vi "GD_GWID5S_info.vi"(8 "error in (no error)":errorcluster, 10 "glue_id":string, 11 "DBlink":string="Driver={ODBC Driver 17 for SQL Server};Server=localhost\\SQLEXPRESS;Database=ZDX201;UID=labview;PWD=Dsa@54137926") -> (0 "error out":errorcluster)   [LabVIEW 2019]
uses:
  <vilib>/addons/database/Connection.llb/DB Tools Open Connec (String).vi
  <vilib>/addons/database/NI_Database_API.lvlib
panel:
  out "Command 2":string="WHERE [id]=13"
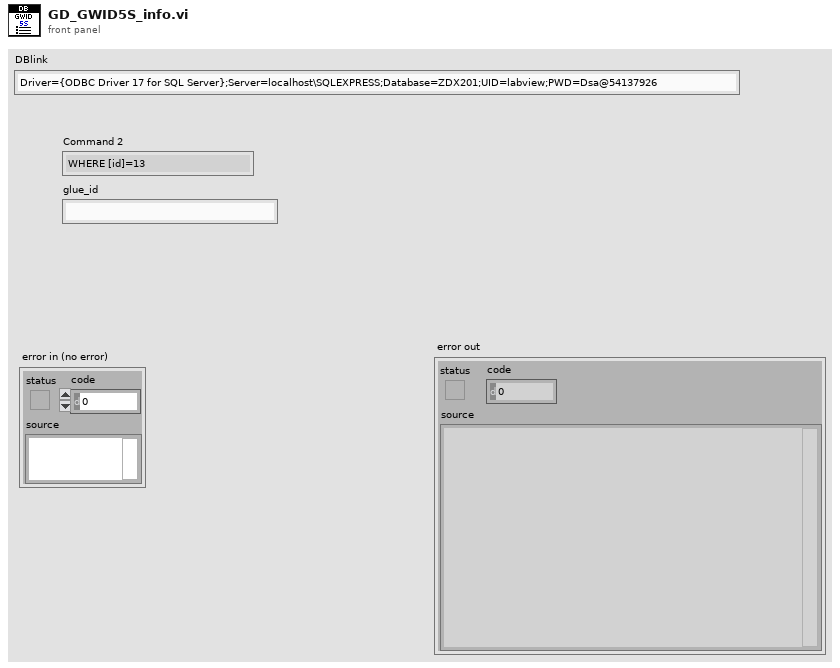
[diagram p1: front panel]
types:
  T1 = cluster{"update_time":timestamp, "eve_time_sb_1":timestamp}
  T2 = typedef "NI_Database_API.lvlib/Conn ObjectReference.ctl" = refnum<k1>
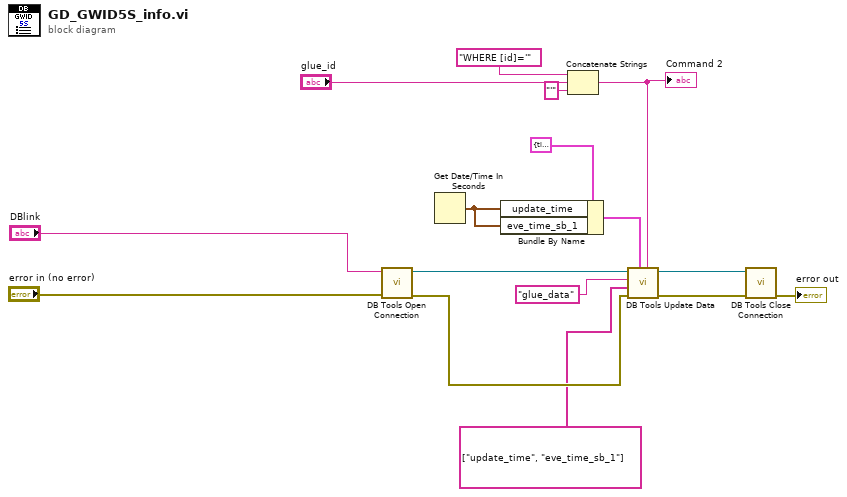
[diagram p0: block diagram]
diagram:
  n1 = call-poly <vilib>:"DB Tools Open Connection.vi"("error in (no error)"="error in (no error)", "connection information"="DBlink") -> ("error out"=w15:errorcluster, "connection reference"=w6:T2)  [unwired: 6 in]
  n2 = Get Date/Time In Seconds() -> (seconds since 1Jan1904=w5:timestamp)
  n3 = Bundle By Name(cluster=T1 {"update_time"=timestamp(0 s since 1904-01-01), "eve_time_sb_1"=timestamp(0 s since 1904-01-01)}, "update_time"=w5, "eve_time_sb_1"=w5) -> (w7:T1)
  n4 = Concatenate Strings("WHERE [id]='", "glue_id", "'" ("string")) -> (w9:string)
  "Command 2" <- w9
  n5 = call <vilib>:"DB Tools Update Data.vi"("condition"=w9, "data"=w7, "error in (no error)"=w15, "columns"=string[] ["update_time", "eve_time_sb_1"], "table"="glue_data", "connection reference"=w6) -> ("error out"=w16:errorcluster, "connection reference out"=w14:T2)  [unwired: 4 in]
  n6 = call <vilib>:"DB Tools Close Connection.vi"("error in (no error)"=w16, "connection reference"=w14) -> ("error out"=→"error out":errorcluster)  [unwired: 5 in]
